vi "Build Tree From Cluster.vi"(7 "Action":T3, 8 "error in":errorcluster, 10 "Display Items":T2(array[cluster]), 11 "Tree Ref":refnum<vi>) -> (0 "error out":errorcluster, 3 "Tree Ref Out":refnum<vi>)   [LabVIEW 2023]
doc: "Take a cluster reference and build a tree of all items in cluster. Set tags of items as \"[row number] item name\" so all tags are unique. Set glyph of its to indicate data type. Set selection color to gray and font size to 18pt."
uses:
  controls/action enum.ctl
panel:
  out "Tree Item Array":T1(array[cluster])
  in  "Tree":string[](tree)
  in  "C1":T4
  # "Debug Cluster"
  # "if display items empty, use this cluster for debug:"
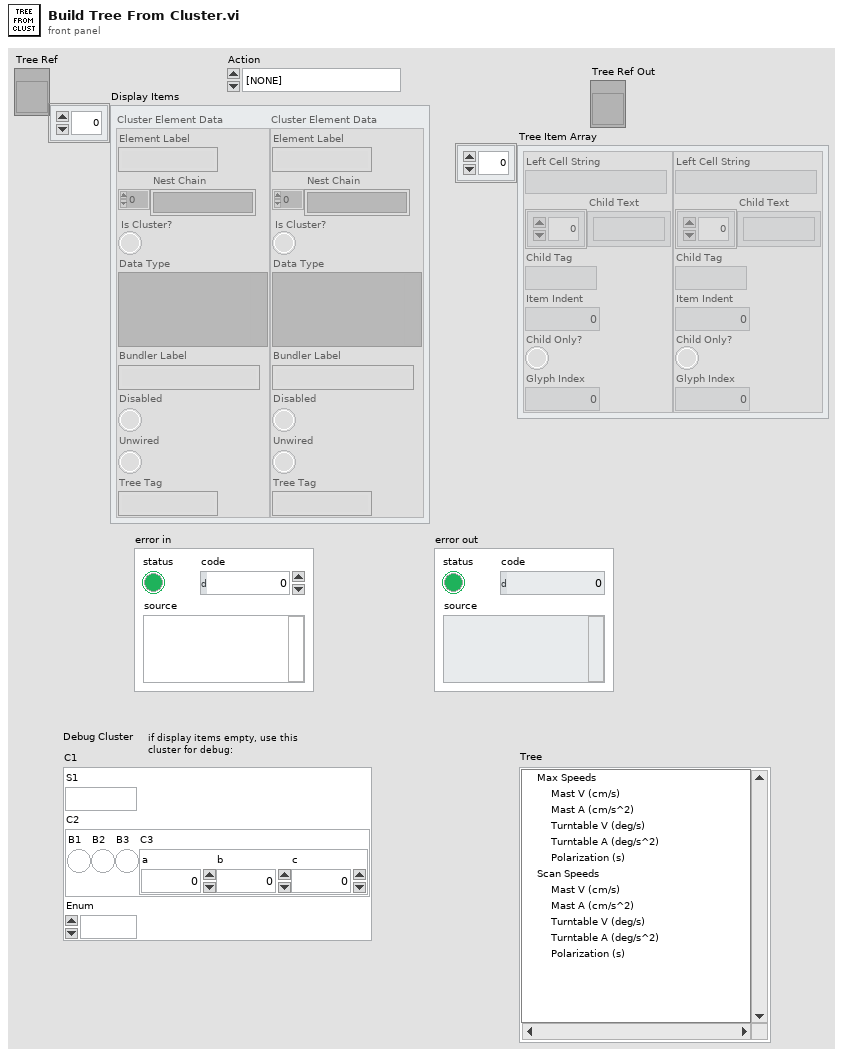
[diagram p1: front panel]
types:
  T1 = cluster{"Left Cell String":string, "Child Text":string[], "Child Tag":string, "Item Indent":i32, "Child Only?":bool, "Glyph Index":i32}[]
  T2 = cluster{"Element Label":string, "Nest Chain":string[], "Is Cluster?":bool, "Data Type":variant, "Bundler Label":string, "Disabled":bool, "Unwired":bool, "Tree Tag":string}[]
  T3 = typedef "action enum.ctl" = enum16{"[NONE]", "Wire Bundle", "Wire Unbundle", "Terminal Unbundle", "Terminal Bundle", "Bundler Move Up", "Bundler Move Down", "Bundler Insert", "Bundler Remove", "Bundler Remove Unwired", "Bundler Rearrange", "In Place Insert", "In Place Remove", "In Place Remove Unwired", "In Place Rearrange", "Wire Properties", "Wire Method", "Terminal Properties", "Terminal Method", "Property Move Up", "Property Move Down", "Properties Insert", "Properties Remove", "Properties Remove Unwired", "Properties Rearrange", "Method Change", "Class for Constant", "Class For Control", "Class For Node", "Class Name to Clipboard"}
  T4 = cluster{"S1":string, "C2":cluster{"B1":bool, "B2":bool, "B3":bool, "C3":cluster{"a":dbl, "b":i32, "c":u8}}, "Enum":enum16{""}}
  T5 = cluster{"image type":i32, "image depth":i32, "image":u8[], "mask":u8[], "colors":u32[], "Rectangle":cluster{"left":i16, "top":i16, "right":i16, "bottom":i16}}
  T6 = typedef "Cluster Element Description.ctl" = cluster{"Element Label":string, "Nest Chain":string[], "Is Cluster?":bool, "Data Type":variant, "Bundler Label":string, "Disabled":bool, "Unwired":bool, "Tree Tag":string}
  T7 = cluster{"left":i16, "top":i16, "right":i16, "bottom":i16}
  T8 = typedef "imagedata.ctl" = cluster{"image type":i32, "image depth":i32, "image":u8[], "mask":u8[], "colors":u32[], "Rectangle":cluster{"left":i16, "top":i16, "right":i16, "bottom":i16}}
  T9 = cluster{"Left Cell String":string, "Child Text":string[], "Child Tag":string, "Item Indent":i32, "Child Only?":bool, "Glyph Index":i32}
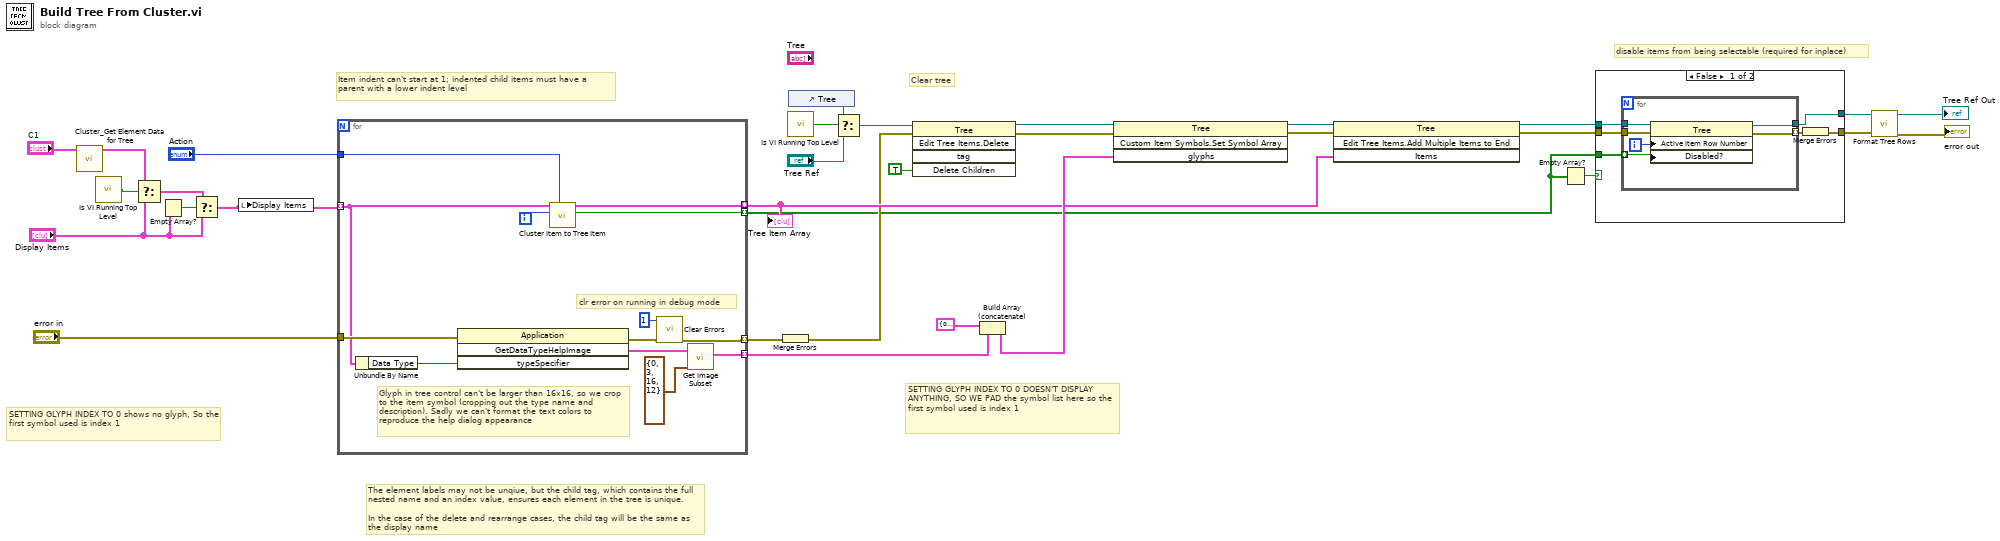
[diagram p0: block diagram]
diagram:
  # "Item indent can't start at 1; indented child items must have a parent with a lower indent level"
  # "Clear tree"
  # "SETTING GLYPH INDEX TO 0 shows no glyph, So the first symbol used is index 1"
  # "disable items from being selectable (required for inplace)"
  # "The element labels may not be unqiue, but the child tag, which contains the full nested name and an index value, ensures each element in the tree is unique. \n\nIn the case of the delete and rearrange cases, the child tag will be the same as the display name"
  # "SETTING GLYPH INDEX TO 0 DOESN'T DISPLAY ANYTHING, SO WE PAD the symbol list here so the first symbol used is index 1"
  n1 = call "Cluster_Get Element Data for Tree.vi"("Data Type"="C1") -> ("Cluster Element Data Aray"=w3:T6[])  [unwired: 10 in]
  n2 = call "Is VI Running Top Level.vi"() -> ("Top Level?"=w18:bool)  [unwired: 5 in]
  n3 = Select(t=w3, s=w18, f="Display Items") -> (s? t:f=w17:T6[])
  n4 = Empty Array?(array="Display Items") -> (empty?=w16:bool)
  n5 = Select(t=w17, s=w16, f="Display Items") -> (s? t:f=w1:T6[])
  n6 = local write "Display Items"(w1) -> ()
  n7 = for {
    tunnel: w1 -> [w34] mode=indexing
    tunnel: [w37] -> w15 mode=indexing
    tunnel: [w43] -> w29 mode=indexing
    tunnel: "Action" -> [w35]
    tunnel: "error in" -> [w41]
    tunnel: [w39] -> w12 mode=indexing
    tunnel: [w36] -> w5 mode=indexing
    i -> [w33]
    # "clr error on running in debug mode"
    # "Glyph in tree control can't be larger than 16x16, so we crop to the item symbol (cropping out the type name and description). Sadly we can't format the text colors to reproduce the help dialog appearance"
    n8 = Unbundle By Name(w34) -> ("Data Type"=w45:variant)
    n9 = invoke class="Application" method="GetDataTypeHelpImage"(error in=w41, "typeSpecifier"=w45) -> (error out=w40:errorcluster, "GetDataTypeHelpImage"=w44:T8)  [unwired: 2 in, 2 out]
    n10 = call "Cluster Item to Tree Item.vi"("Action"=w35, "Index"=w33, "Cluster Element Data"=w34) -> ("Disable"=w36:bool, "Item"=w37:T9)  [unwired: 7 in]
    n11 = call <vilib>:"Clear Errors.vi"("error in (no error)"=w40, "specific error code to clear (0: all)"=1) -> ("error out"=w39:errorcluster)  [unwired: 4 in, 1 out]
    n12 = call <vilib>:"Get Image Subset.vi"("subset rect"=T7 {"left"=0, "top"=3, "right"=16, "bottom"=12}, "image data"=w44) -> ("image subset"=w43:T8)  [unwired: 4 in, 1 out]
  }
  "Tree Item Array" <- w15
  n13 = Merge Errors(w12) -> (w11:errorcluster)
  n14 = call "Is VI Running Top Level.vi"() -> ("Top Level?"=w27:bool)  [unwired: 5 in]
  n15 = control-ref of="Tree"() -> (w25:refnum<vi>)
  n16 = Select(t=w25, s=w27, f="Tree Ref") -> (s? t:f=w24:refnum<vi>)
  n17 = invoke class="Tree" method="Edit Tree Items.Delete"(reference=w24, error in=w11, "Delete Children"=TRUE ("Delete Children?")) -> (reference out=w22:refnum<vi>, error out=w21:errorcluster)  [unwired: 2 in, 3 out]
  n18 = Build Array (concatenate)(T5 {"image type"=0, "image depth"=0, "image"=[], "mask"=[], "colors"=[], "Rectangle"={"left"=0, "top"=0, "right"=0, "bottom"=0}} ("image subset"), w29) -> (w28:T8[])
  n19 = invoke class="Tree" method="Custom Item Symbols.Set Symbol Array"(reference=w22, error in=w21, "glyphs"=w28) -> (reference out=w31:refnum<vi>, error out=w23:errorcluster)  [unwired: 1 in, 2 out]
  n20 = invoke class="Tree" method="Edit Tree Items.Add Multiple Items to End"(reference=w31, error in=w23, "Items"=w15) -> (reference out=w20:refnum<vi>, error out=w19:errorcluster)  [unwired: 1 in, 2 out]
  n21 = Empty Array?(array=w5) -> (empty?=w7:bool)
  n22 = case shown="False" w7 {
    tunnel: w20 -> [w51 w59]
    tunnel: w19 -> [w50 w58]
    tunnel: w5 -> [w48 _]
    tunnel: [w47 w58] -> w10
    tunnel: [w46 w59] -> w9
    frame False {
      n23 = for {
        tunnel: w48 -> [w53] mode=indexing
        tunnel: w50 -> [w56]
        tunnel: [w54] -> w49 mode=indexing
        tunnel: w51 -> [w57]
        tunnel: [w55] -> w46
        i -> [w52]
        n24 = property class="Tree"(reference=w57, error in=w56, "Active Item Row Number"=w52, "Disabled?"=w53) -> (reference out=w55:refnum<vi>, error out=w54:errorcluster)
      }
      n25 = Merge Errors(w49) -> (w47:errorcluster)
    }
    frame True {
    }
  }
  n26 = call "Format Tree Rows.vi"("error in"=w10, "Tree Ref"=w9) -> ("error out"=→"error out":errorcluster, "Tree Ref out"=→"Tree Ref Out":refnum<vi>)  [unwired: 8 in]
